vi "Cache-BroadcastReg Status of Source.vi"(8 "error in (no error)":errorcluster, 10 "CSM Name":string, 11 "Broadcast State":string) -> (0 "error out":errorcluster, 1 "State Matched":bool)   [LabVIEW 2017, in "Communicable State Machine.lvlib"]
uses:
  Communicable State Machine.lvlib
  Typedef/_CSM_List Module Scope.ctl
  Operation-BroadcastRegistry.ctl
  ChangeFlag/ChangeFlag-Read.vi
  ChangeFlag/ChangeFlagDB.vi
  AdvanceAPI/CSM - Broadcast Message Type.ctl
  _Shared/CSM Shared.lvlib
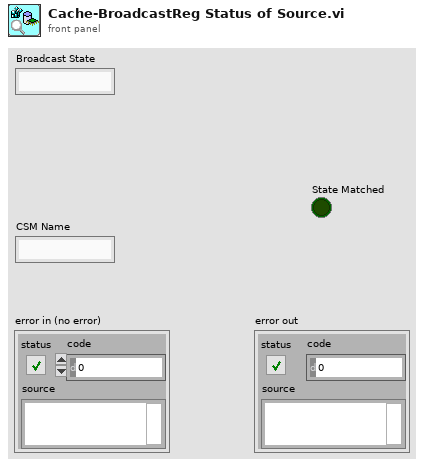
[diagram p1: front panel]
types:
  T1 = typedef "Communicable State Machine.lvlib/_CSM_List Module Scope.ctl" = enum16{"Normal", "System Only", "All"}
  T2 = typedef "Communicable State Machine.lvlib/Operation-BroadcastRegistry.ctl" = enum16{"Delete Source Module", "Delete Target Module", "Remove Module", "Register", "Unregister", "Check", "List Status", "List Entries", "List Status Of Source"}
  T3 = typedef "Communicable State Machine.lvlib/CSM - Broadcast Message Type.ctl" = enum16{"Status", "Interrupt(High)"}
  T4 = cluster{"Target CSM":string, "Target State":string, "Priority":T3}
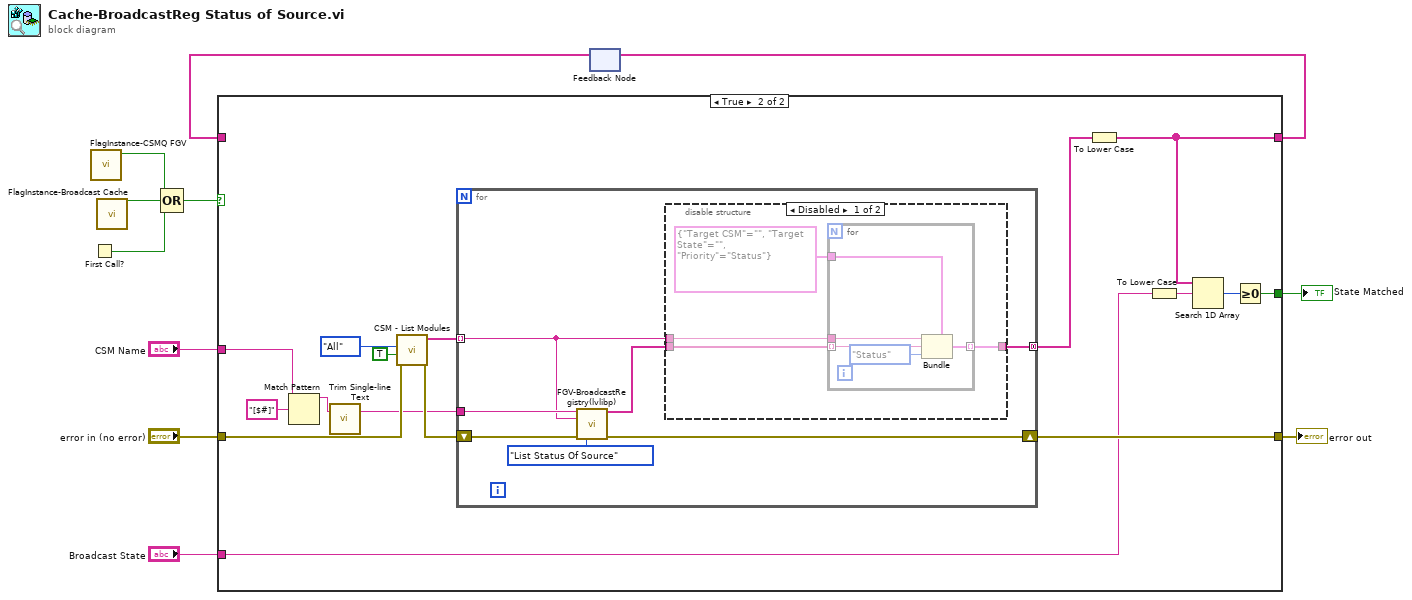
[diagram p0: block diagram]
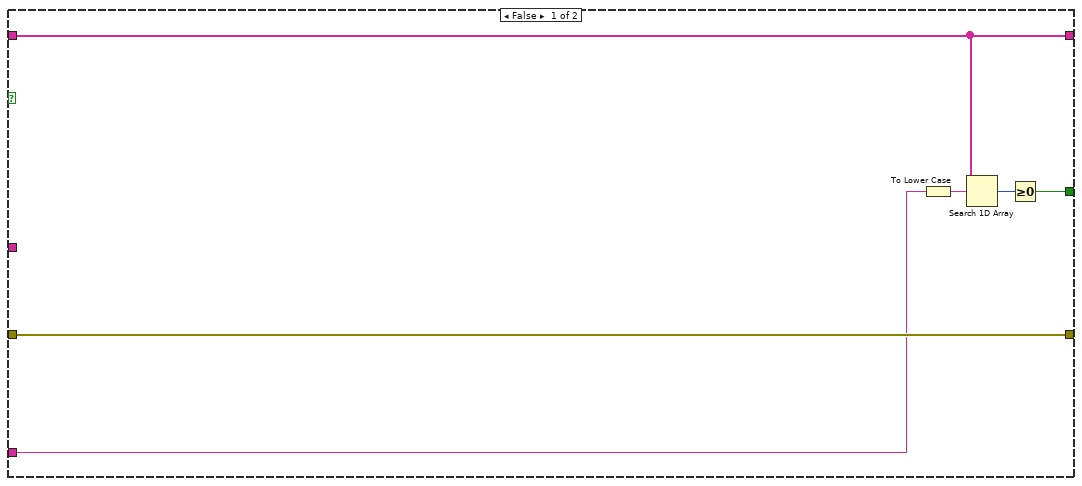
[diagram p2: hidden frame]
diagram:
  n1 = First Call?() -> (First Call?: T/F=w9:bool)
  n2 = call "FlagInstance-CSMQ FGV.vi"() -> ("Changed"=w2:bool)  [unwired: 10 in, 1 out]
  n3 = call "FlagInstance-Broadcast Cache.vi"() -> ("Changed"=w1:bool)  [unwired: 10 in, 1 out]
  n4 = Compound Arithmetic op=OR(w2, w1, w9) -> (w5:bool)
  n5 = feedback #1() -> (w6:string[])  [unwired: 1 in]
  n6 = case shown="True" w5 {
    tunnel: [w17 w33] -> w11
    tunnel: "error in (no error)" -> [w17 w31]
    tunnel: "Broadcast State" -> [w15 w18]
    tunnel: [w16 w19] -> w8
    tunnel: w6 -> [w16 _]
    tunnel: "CSM Name" -> [_ w25]
    tunnel: [w13 w20] -> w3
    frame False {
      n7 = To Lower Case(string=w15) -> (all lower case string=w12:string)
      n8 = Search 1D Array(1D array=w16, element=w12) -> (index of element=w14:i32)  [unwired: 1 in]
      n9 = Greater Or Equal To 0?(x=w14) -> (x >= 0?=w13:bool)
    }
    frame True {
      n10 = Match Pattern(string=w25, regular expression="[$#]") -> (before substring=w26:string)  [unwired: 1 in, 3 out]
      n11 = call "Trim Single-line Text.vi"("single-line text"=w26) -> ("trimed text"=w23:string)  [unwired: 2 in]
      n12 = call "CSM - List Modules.vi"("Error In"=w31, "With Instance? (F)"=TRUE ("With Instance(F)"), "Scope (Normal)"=_CSM_List_Module_Scope."All" ("Scope(Normal)")) -> ("error out"=w32:errorcluster, "Module Names"=w30:string[])  [unwired: 7 in]
      n13 = for {
        tunnel: w23 -> [w38]
        shift-right: [w37] -> w33
        shift-left: w32 -> [w39]
        tunnel: [w36] -> w27 mode=concatenating
        tunnel: w30 -> [w34] mode=indexing
        n14 = call "FGV-BroadcastRegistry(lvlibp).vi"("Source"=w38, "Target"=w34, "Error In"=w39, "Operation"=Operation-BroadcastRegistry."List Status Of Source") -> ("Response Message"=w35:string[], "error out"=w37:errorcluster)  [unwired: 10 in]
        n15 = disable-structure shown="Disabled" {
          disable-tunnel: [w44 w50] -> w36
          disable-tunnel: w35 -> [w43 w50]
          disable-tunnel: w34 -> [w42 _]
          frame Disabled {
            n16 = for {
              tunnel: w42 -> [w47]
              tunnel: T4 {"Target CSM"="", "Target State"="", "Priority"=enum."Status"} ("cluster") -> [w48]
              tunnel: [w49] -> w44 mode=indexing
              tunnel: w43 -> [w46] mode=indexing
              n17 = Bundle(cluster=w48, "Target CSM"=w47, "Target State"=w46, "Priority"=CSM_-_Broadcast_Message_Type."Status") -> (w49:T4)
            }
          }
          frame Enabled {
          }
        }
      }
      n18 = To Lower Case(string=w27) -> (all lower case string=w19:string[])
      n19 = To Lower Case(string=w18) -> (all lower case string=w21:string)
      n20 = Search 1D Array(1D array=w19, element=w21) -> (index of element=w22:i32)  [unwired: 1 in]
      n21 = Greater Or Equal To 0?(x=w22) -> (x >= 0?=w20:bool)
    }
  }
  "error out" <- w11
  "State Matched" <- w3
  n22 = feedback-in #1(w8) -> ()
